vi "__rotateBuffer.vi"(0 "data in":dbl[](array[numeric]), 1 "new parameter":dbl) -> (20 "data out":dbl[](array[numeric]))   [LabVIEW 2020, in "BME280.lvclass"]
uses:
  BME280.lvclass
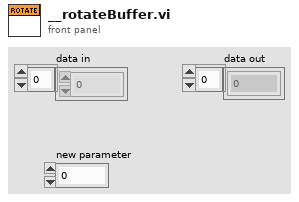
[diagram p1: front panel]
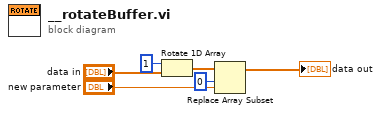
[diagram p0: block diagram]
diagram:
  n1 = Rotate 1D Array(1:"data in", 2:1 ("n")) -> (0:w3:dbl[])
  n2 = Replace Array Subset(array=w3, new element="new parameter", index=0) -> (→"data out":dbl[])
